vi "XYZOAT to T.vi"(9 "XYZOAT":T1) -> (1 "T":T2 format="%.3f")   [LabVIEW 2013]
uses:
  <vilib>/Analysis/Matrix/Datatypes/RealMatrix.ctl
  <vilib>/Analysis/Matrix/Numeric/Conversions/Array To Matrix - RA2.vi
  <vilib>/Analysis/Matrix/Numeric/Multiply/Multiply - RM,RM.vi
  <vilib>/Analysis/Matrix/NI_Matrix.lvlib
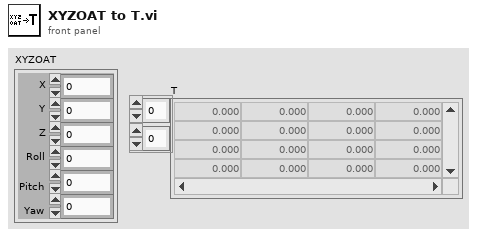
[diagram p1: front panel]
types:
  T1 = cluster{"X":dbl, "Y":dbl, "Z":dbl, "Roll":dbl, "Pitch":dbl, "Yaw":dbl}
  T2 = typedef "NI_Matrix.lvlib/RealMatrix.ctl" = dbl[][]
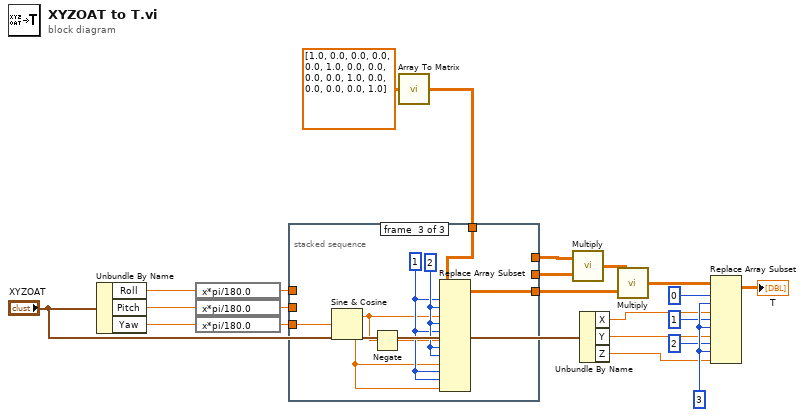
[diagram p0: block diagram]
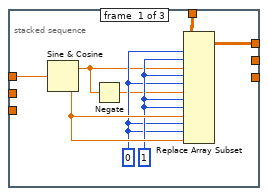
[diagram p2: hidden frame]
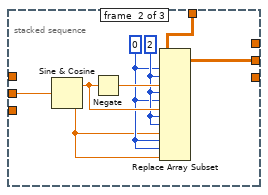
[diagram p3: hidden frame]
diagram:
  w14 = 3 ("disabled index (col)")
  n1 = Unbundle By Name("XYZOAT") -> ("Roll"=w7:dbl, "Pitch"=w6:dbl, "Yaw"=w5:dbl)
  n2 = expression code="x*pi/180.0" ("radians to degrees")(w7) -> (w10:dbl)
  n3 = expression code="x*pi/180.0" ("radians to degrees")(w6) -> (w9:dbl)
  n4 = expression code="x*pi/180.0" ("radians to degrees")(w5) -> (w8:dbl)
  n5 = call-poly <vilib>:"Array To Matrix.vi"("Real 2D Array"=dbl[][] [[1.0, 0.0, 0.0, 0.0], [0.0, 1.0, 0.0, 0.0], [0.0, 0.0, 1.0, 0.0], [0.0, 0.0, 0.0, 1.0]]) -> ("Real Matrix"=w21:T2)
  n6 = stacked-sequence {
    tunnel: w21 -> [w30 w38 w46]
    tunnel: [w29 _ _] -> w20
    tunnel: w9 -> [_ w31 _]
    tunnel: [_ w37 _] -> w19
    tunnel: w8 -> [_ _ w41]
    tunnel: [_ _ w42] -> w17
    tunnel: w10 -> [w25 _ _]
    frame #0 {
      w27 = 1 ("index (row)")
      w26 = 0 ("index (row)")
      n7 = Sine & Cosine(0:w25) -> (1:w24:dbl, 2:w28:dbl)
      n8 = Negate(x=w24) -> (-x=w23:dbl)
      n9 = Replace Array Subset(array=w30, new element #1=w24, index (row) #1=w26, index (col) #1=w27, new element #2=w23, index (row) #2=w27, index (col) #2=w26, new element #3=w28, index (row) #3=w27, index (col) #3=w27, new element #4=w28, index (row) #4=w26, index (col) #4=w26) -> (w29:T2)
    }
    frame #1 {
      w33 = 0 ("index (row)")
      w34 = 2 ("index (row)")
      n10 = Sine & Cosine(0:w31) -> (1:w35:dbl, 2:w32:dbl)
      n11 = Negate(x=w35) -> (-x=w36:dbl)
      n12 = Replace Array Subset(array=w38, new element #1=w36, index (row) #1=w33, index (col) #1=w34, new element #2=w35, index (row) #2=w34, index (col) #2=w33, new element #3=w32, index (row) #3=w34, index (col) #3=w34, new element #4=w32, index (row) #4=w33, index (col) #4=w33) -> (w37:T2)
    }
    frame #2 {
      w44 = 1 ("index (row)")
      w45 = 2 ("index (row)")
      n13 = Sine & Cosine(0:w41) -> (1:w40:dbl, 2:w43:dbl)
      n14 = Negate(x=w40) -> (-x=w39:dbl)
      n15 = Replace Array Subset(array=w46, new element #1=w40, index (row) #1=w44, index (col) #1=w45, new element #2=w39, index (row) #2=w45, index (col) #2=w44, new element #3=w43, index (row) #3=w45, index (col) #3=w45, new element #4=w43, index (row) #4=w44, index (col) #4=w44) -> (w42:T2)
    }
  }
  n16 = call-poly <vilib>:"Multiply.vi"("Real Matrix B"=w19, "Real Matrix A"=w20) -> ("A * B"=w18:T2)
  n17 = Unbundle By Name("XYZOAT") -> ("X"=w4:dbl, "Y"=w3:dbl, "Z"=w2:dbl)
  n18 = call-poly <vilib>:"Multiply.vi"("Real Matrix B"=w17, "Real Matrix A"=w18) -> ("A * B"=w16:T2)
  n19 = Replace Array Subset(array=w16, new element #1=w4, index (row) #1=0 ("disabled index (row)"), index (col) #1=w14, new element #2=w3, index (row) #2=1 ("disabled index (row)"), index (col) #2=w14, new element #3=w2, index (row) #3=2 ("disabled index (row)"), index (col) #3=w14) -> (→"T":T2)
